vi "GV pixel clock count.vi"() -> ()   [LabVIEW 2017]
panel:
  out "Pixel clock count":u16
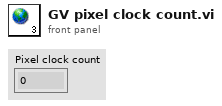
[diagram p1: front panel]
diagram:
